vi "Output.vi"   [LabVIEW 2017, in "HD44780 Host.lvlib"]
doc: "Writes text strings or character codes on character LCD devices."
uses:
  HD44780 Host.lvlib
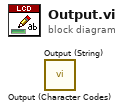
[diagram p0: block diagram]
diagram:
  n1 = call "Output (Character Codes).vi"() -> ()  [unwired: 9 in, 3 out]
  n2 = call "Output (String).vi"() -> ()  [unwired: 9 in, 3 out]
